vi "Model Parameter List.vi"(1 "Fit Model":T2) -> (0 "Model Parameter List":T1[](array[typedef]))   [LabVIEW 2021, in "Fits.lvlib"]
uses:
  Fits.lvlib
  Decay Model.ctl
  IRF(X)PSED/Decay Fit Parameters In List.ctl
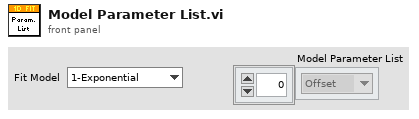
[diagram p1: front panel]
types:
  T1 = typedef "Fits.lvlib/Decay Fit Parameters In List.ctl" = enum16{"Offset", "Baseline", "A_1", "tau_1", "A_2", "tau_2"}
  T2 = typedef "Fits.lvlib/Decay Model.ctl" = enum16{"1-Exponential", "2-Exponentials"}
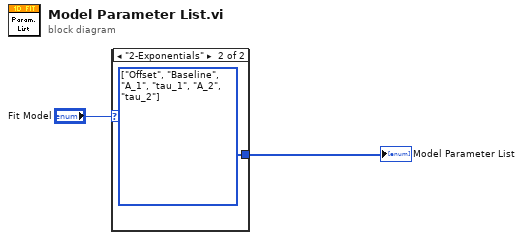
[diagram p0: block diagram]
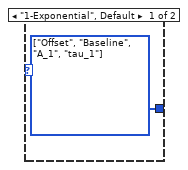
[diagram p2: hidden frame]
diagram:
  n1 = case shown="\"2-Exponentials\"" "Fit Model" {
    tunnel: [w3 w4] -> w1
    frame "1-Exponential", Default {
      w3 = T1[] [enum."Offset", enum."Baseline", enum."A_1", enum."tau_1"] items=["Offset", "Baseline", "A_1", "tau_1", "A_2", "tau_2"] ("Array")
    }
    frame "2-Exponentials" {
      w4 = T1[] [enum."Offset", enum."Baseline", enum."A_1", enum."tau_1", enum."A_2", enum."tau_2"] items=["Offset", "Baseline", "A_1", "tau_1", "A_2", "tau_2"] ("Array")
    }
  }
  "Model Parameter List" <- w1
